vi "sendEventToClient.vi"(8 "error in (no error)":errorcluster, 11 "TcpServer out":refnum<class "TcpServer.lvclass">) -> (0 "error out":errorcluster, 3 "tcpServer out":refnum<class "TcpServer.lvclass">)   [LabVIEW 2018]
doc: "Send an event to the TCP client."
uses:
  src/TcpServer/TcpServer.lvclass
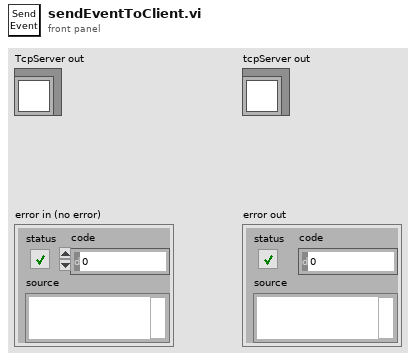
[diagram p1: front panel]
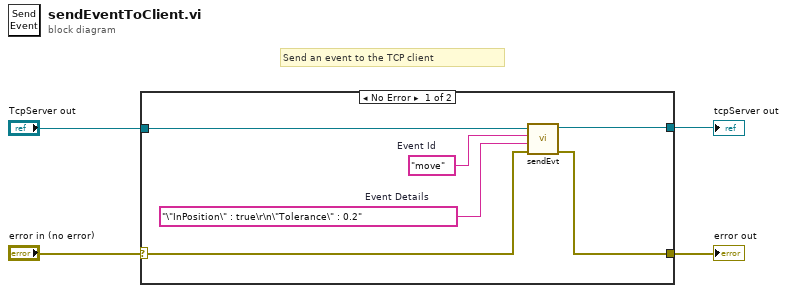
[diagram p0: block diagram]
diagram:
  # "Send an event to the TCP client"
  n1 = case shown="No Error" "error in (no error)" {
    selector: "error in (no error)" -> [w9 w11]
    tunnel: "TcpServer out" -> [w10 w12]
    tunnel: [w8 w12] -> w2
    tunnel: [w7 w11] -> w1
    frame No Error {
      w5 = "\"InPosition\" : true\r\n\"Tolerance\" : 0.2"  # Event Details
      w6 = "move"  # Event Id
      n2 = call "sendEvt.vi"("error in (no error)"=w9, "Event Details"=w5, "Event Id"=w6, "tcpServer in"=w10) -> ("error out"=w7:errorcluster, "tcpServer out"=w8:refnum<class "TcpServer.lvclass">)  [unwired: 6 in]
    }
    frame Error {
    }
  }
  "error out" <- w1
  "tcpServer out" <- w2
